vi "Pre Launch Init.vi"(11 "Generador de Funciones in":refnum<class "Generador de Funciones.lvclass">) -> (0 "error out":errorcluster, 3 "Generador de Funciones out":refnum<class "Generador de Funciones.lvclass">)   [LabVIEW 2020, in "Generador de Funciones.lvlib" / "Generador de Funciones.lvclass"]
doc: "(<B>Filename</B>: Actor Framework.lvlib:Actor.lvclass:Pre Launch Init.vi)\n\nDefines behavior that occurs after the Launch Nested Actor method is invoked but before the actor's Actor Core method begins running.\n\nBy default, this method does nothing. A descendant class may override it to define behavior."
uses:
  Generador de Funciones.lvclass
  Generador de Funciones.lvclass/Generador de Funciones.ctl
  <vilib>/ActorFramework/Actor/Actor.lvclass
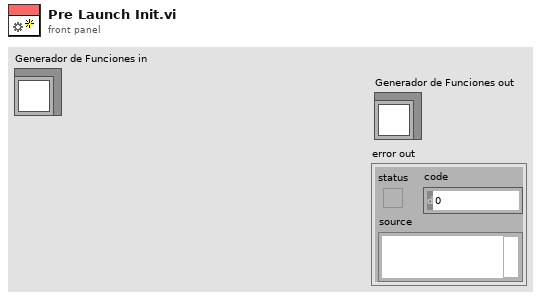
[diagram p1: front panel]
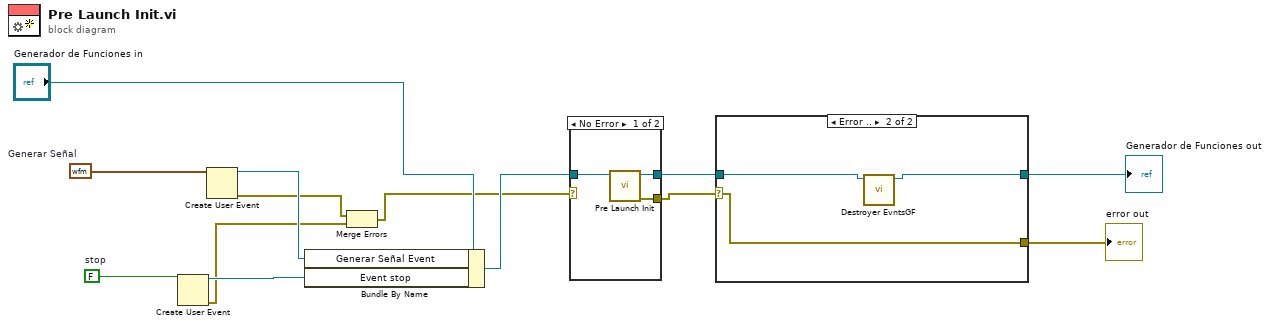
[diagram p0: block diagram]
diagram:
  w12 = FALSE  # stop
  w13 = waveform(dbl) {"t0"=timestamp(0 s since 1904-01-01), "dt"=1.0, "Y"=[]}  # Generar Señal
  n1 = Create User Event(user event datatype=w12) -> (user event=w9:refnum<user-event>, error out=w6:errorcluster)  [unwired: 1 in]
  n2 = Create User Event(user event datatype=w13) -> (user event=w8:refnum<user-event>, error out=w7:errorcluster)  [unwired: 1 in]
  n3 = Bundle By Name(cluster="Generador de Funciones in", "Generar Señal Event"=w8, "Event stop"=w9) -> (w10:refnum<class "Generador de Funciones.lvclass">)
  n4 = Merge Errors(w7, w6) -> (w5:errorcluster)
  n5 = case shown="No Error" w5 {
    selector: w5 -> [_ w17]
    tunnel: [w16 w17] -> w4
    tunnel: [w15 w18] -> w3
    tunnel: w10 -> [w14 w18]
    frame No Error {
      n6 = call-parent "Pre Launch Init.vi"("Actor in"=w14) -> ("error out"=w16:errorcluster, "Actor out"=w15:refnum<class "Generador de Funciones.lvclass">)  [unwired: 9 in]
    }
    frame Error {
    }
  }
  n7 = case shown="Error .." w4 {
    selector: w4 -> [w19 w23]
    tunnel: w3 -> [w20 w21]
    tunnel: [w20 w22] -> w2
    tunnel: [w19 w23] -> w1
    frame No Error {
    }
    frame Error {
      n8 = call "Destroyer EvntsGF.vi"("Generador de Funciones in"=w21) -> ("Generador de Funciones out"=w22:refnum<class "Generador de Funciones.lvclass">)  [unwired: 10 in]
    }
  }
  "error out" <- w1
  "Generador de Funciones out" <- w2
